vi "Initialize.vi"(8 "error in (no error)":errorcluster, 9 "Reset (True)":bool=TRUE, 10 "ID Query (True)":bool=TRUE, 11 "VISA resource name":refnum<visa-resource-name>) -> (0 "error out":errorcluster, 3 "VISA resource name out":refnum<visa-resource-name>)   [LabVIEW 2020, in "Agilent 3446X Series.lvlib"]
doc: "Establishes communication with the instrument and optionally performs an instrument identification query and/or an instrument reset. It also places the instrument in a default state needed for other instrument driver operations. Therefore, call this VI before calling other instrument driver VIs for this instrument. Generally, you need to call the Initialize VI only once at the beginning of an application."
uses:
  <instrlib>/Agilent 3446X Series/Agilent 3446X Series.lvlib
  <vilib>/regexp/Match Regular Expression.xnode
panel:
  # "(c) 2013-2021 National Instruments.  ALL RIGHTS RESERVED."
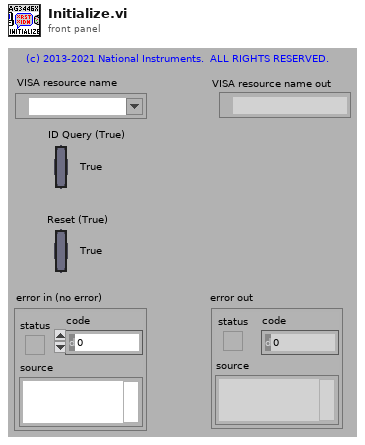
[diagram p1: front panel]
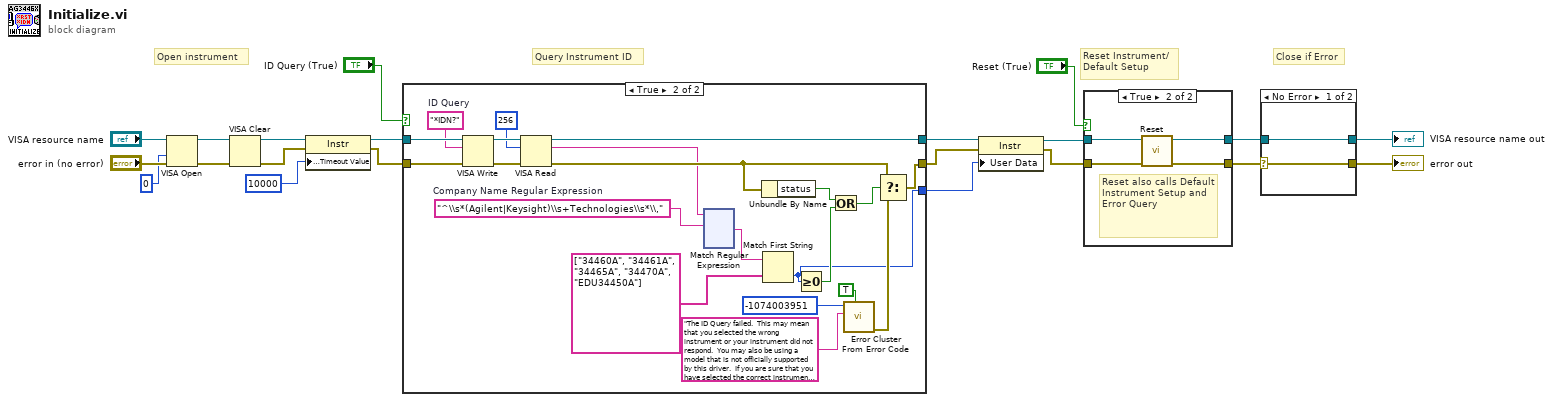
[diagram p0: block diagram]
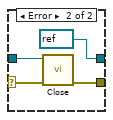
[diagram p2: hidden frame]
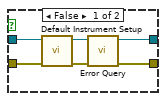
[diagram p3: hidden frame]
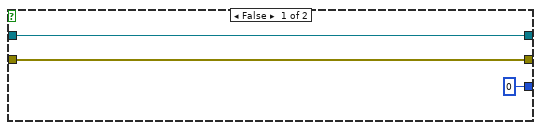
[diagram p4: hidden frame]
diagram:
  # "Close if Error"
  # "Query Instrument ID"
  # "Reset Instrument/\nDefault Setup"
  # "Open instrument"
  n1 = VISA Open(access mode=u32 0, error in (no error)="error in (no error)", VISA resource name="VISA resource name") -> (VISA resource name=w15:refnum<visa-resource-name>, error out=w14:errorcluster)  [unwired: 2 out]
  n2 = VISA Clear(VISA resource name=w15, error in (no error)=w14) -> (VISA resource name out=w13:refnum<visa-resource-name>, error out=w12:errorcluster)
  n3 = property class="Instr"(reference=w13, error in=w12, "General Settings:Timeout Value"=u32 10000) -> (reference out=w7:refnum<visa-resource-name>, error out=w6:errorcluster)
  n4 = case shown="True" "ID Query (True)" {
    tunnel: [w23 w45] -> w3
    tunnel: [w24 w42] -> w5
    tunnel: w7 -> [w24 w43]
    tunnel: w6 -> [w23 w44]
    tunnel: [0 ("Code") w25] -> w1
    frame False {
    }
    frame True {
      w29 = "^\\s*(Agilent|Keysight)\\s+Technologies\\s*\\,"  # Company Name Regular Expression
      w38 = "*IDN?"  # ID Query
      n5 = VISA Write(VISA resource name=w43, write buffer=w38, error in (no error)=w44) -> (VISA resource name out=w41:refnum<visa-resource-name>, error out=w40:errorcluster)  [unwired: 1 out]
      n6 = VISA Read(VISA resource name=w41, byte count=u32 256, error in (no error)=w40) -> (VISA resource name out=w42:refnum<visa-resource-name>, read buffer=w28:string, error out=w34:errorcluster)  [unwired: 1 out]
      n7 = xnode "Match Regular Expression"("input string"=w28, "regular expression"=w29) -> ("after match"=w27:string)  [unwired: 4 in, 4 out]
      n8 = Unbundle By Name(w34) -> ("status"=w33:bool)
      n9 = Match First String(2:string[] ["34460A", "34461A", "34465A", "34470A", "EDU34450A"] ("string array"), 3:w27) -> (0:w25:i32)  [unwired: 1 out]
      n10 = Greater Or Equal To 0?(x=w25) -> (x >= 0?=w32:bool)
      n11 = Or(x=w33, y=w32) -> (x .or. y?=w31:bool)
      n12 = call <vilib>:"Error Cluster From Error Code.vi"("show call chain? (False)"=TRUE, "error message (\"\")"="The ID Query failed.  This may mean that you selected the wrong instrument or your instrument did not respond.  You may also be using a model that is not officially supported by this driver.  If you are sure that you have selected the correct instrument and it is responding, try disabling the ID Query." ("Source (VI Name)"), "error code (0)"=-1074003951 ("Code")) -> ("error out"=w37:errorcluster)  [unwired: 1 in, 5 out]
      n13 = Select(t=w34, s=w31, f=w37) -> (s? t:f=w45:errorcluster)
    }
  }
  n14 = property class="Instr"(reference=w5, error in=w3, "User Data"=w1) -> (reference out=w4:refnum<visa-resource-name>, error out=w2:errorcluster)
  n15 = case shown="True" "Reset (True)" {
    tunnel: w2 -> [w164 w166]
    tunnel: [w161 w169] -> w8
    tunnel: w4 -> [w165 w167]
    tunnel: [w162 w168] -> w9
    frame False {
      n16 = call <instrlib>:"Default Instrument Setup.vi"("error in (no error)"=w164, "VISA resource name"=w165) -> ("error out"=w160:errorcluster, "VISA resource name out"=w163:refnum<visa-resource-name>)  [unwired: 8 out]
      n17 = call <instrlib>:"Error Query.vi"("error in (no error)"=w160, "VISA resource name"=w163) -> ("error out"=w161:errorcluster, "VISA resource name out"=w162:refnum<visa-resource-name>)  [unwired: 8 out]
    }
    frame True {
      # "Reset also calls Default Instrument Setup and Error Query"
      n18 = call <instrlib>:"Reset.vi"("error in (no error)"=w166, "VISA resource name"=w167) -> ("error out"=w169:errorcluster, "VISA resource name out"=w168:refnum<visa-resource-name>)  [unwired: 8 out]
    }
  }
  n19 = case shown="No Error" w8 {
    selector: w8 -> [w170 w173]
    tunnel: w9 -> [w171 w174]
    tunnel: [w171 refnum<visa-resource-name> refnum ("VISA resource name out")] -> w11
    tunnel: [w170 w175] -> w10
    frame No Error {
    }
    frame Error {
      n20 = call <instrlib>:"Close.vi"("error in (no error)"=w173, "VISA resource name"=w174) -> ("error out"=w175:errorcluster)  [unwired: 9 out]
    }
  }
  "VISA resource name out" <- w11
  "error out" <- w10
